vi "Write EEPROM.vi"(8 "error in (no error)":errorcluster, 9 "Offset":u8, 10 "Data":u8[](array[numeric]), 11 "RTL-SDR in":refnum<class "RTL-SDR.lvclass">) -> (0 "error out":errorcluster, 1 "function return":i32, 2 "Length":u16, 3 "RTL-SDR out":refnum<class "RTL-SDR.lvclass">)   [LabVIEW 2015, in "RTL-SDR.lvclass"]
doc: "Created IvanLis by LabVIEW Portal\nProfile: http://labviewportal.org/memberlist.php?mode=viewprofile&u=987\neMail: IvanLisanov@gMail.com\nTelegram: https://t.me/IvanLis"
uses:
  RTL-SDR.lvclass
  RTL-SDR.lvclass/RTL-SDR.ctl
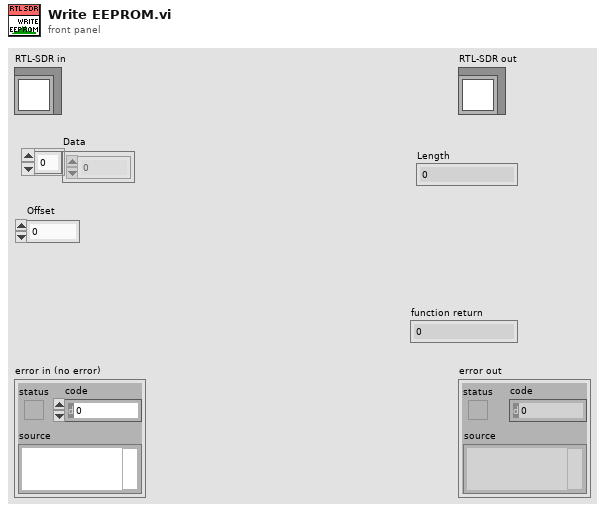
[diagram p1: front panel]
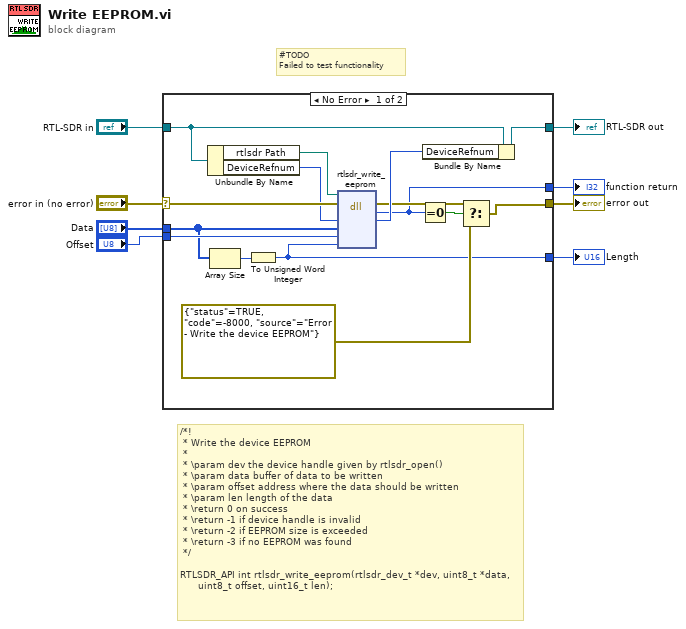
[diagram p0: block diagram]
diagram:
  # "#TODO\nFailed to test functionality"
  # "/*!\n * Write the device EEPROM\n *\n * \\param dev the device handle given by rtlsdr_open()\n * \\param data buffer of data to be written\n * \\param offset address where the data should be written\n * \\param len length of the data\n * \\return 0 on success\n * \\return -1 if device handle is invalid\n * \\return -2 if EEPROM size is exceeded\n * \\return -3 if no EEPROM was found\n */\n\nRTLSDR_API int rtlsdr_write_eeprom(rtlsdr_dev_t *dev, uint8_t *data,\n\t\t\t\t  uint8_t offset, uint16_t len);"
  n1 = case shown="No Error" "error in (no error)" {
    selector: "error in (no error)" -> [w23 w25]
    tunnel: [w13 w25] -> w7
    tunnel: [w21 w24] -> w5
    tunnel: "RTL-SDR in" -> [w22 w24]
    tunnel: [w12 _] -> w4
    tunnel: "Data" -> [w11 _]
    tunnel: "Offset" -> [w17 _]
    tunnel: [w9 _] -> w1
    frame No Error {
      n2 = Unbundle By Name(w22) -> ("rtlsdr Path"=w20:path, "DeviceRefnum"=w19:u64)
      n3 = Array Size(array=w11) -> (size(s)=w10:i32)
      n4 = To Unsigned Word Integer(number=w10) -> (unsigned 16bit integer=w9:u16)
      n5 = dll-call lib="C:/Users/Ivan/Desktop/RTL-SDR Class/Project (RTL-SDR)/RTL-SDR Class/dll/rtlsdr.dll" fn="rtlsdr_write_eeprom"(path in=w20, error in=w23, "DeviceRefnum"=w19, "Data"=w11, "Offset"=w17, "Length"=w9) -> (error out=w14:errorcluster, "return type"=w12:i32, "DeviceRefnum"=w18:u64)  [unwired: 4 in, 1 out]
      n6 = Equal To 0?(x=w12) -> (x = 0?=w15:bool)
      n7 = Bundle By Name(cluster=w22, "DeviceRefnum"=w18) -> (w21:refnum<class "RTL-SDR.lvclass">)
      n8 = Select(t=w14, s=w15, f=errorcluster {"status"=TRUE, "code"=-8000, "source"="Error - Write the device EEPROM"} ("error out")) -> (s? t:f=w13:errorcluster)
    }
    frame Error {
    }
  }
  "error out" <- w7
  "RTL-SDR out" <- w5
  "function return" <- w4
  "Length" <- w1
